vi "q2 binary to decimal.vi"() -> ()   [LabVIEW 2025]
panel:
  out "decimal":dbl
  in  "position 1":dbl
  in  "position 3":dbl
  in  "position 2":dbl
  in  "position 0":dbl
  in  "b0":bool
  in  "b1":bool
  in  "b2":bool
  in  "b3":bool
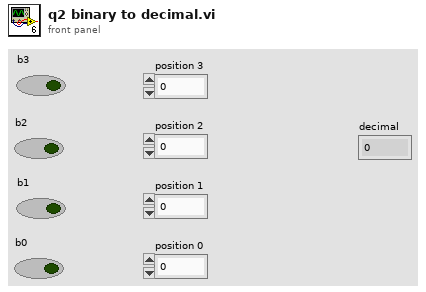
[diagram p1: front panel]
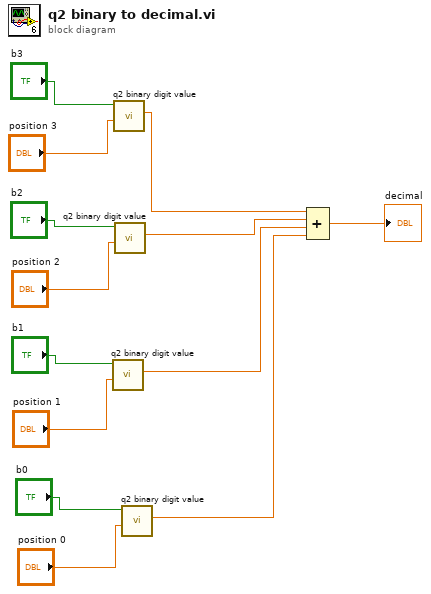
[diagram p0: block diagram]
diagram:
  n1 = call "q2 binary digit value.vi"("position"="position 1", "b"="b1") -> ("value"=w3:dbl)  [unwired: 9 in]
  n2 = call "q2 binary digit value.vi"("position"="position 3", "b"="b3") -> ("value"=w5:dbl)  [unwired: 9 in]
  n3 = call "q2 binary digit value.vi"("position"="position 2", "b"="b2") -> ("value"=w4:dbl)  [unwired: 9 in]
  n4 = call "q2 binary digit value.vi"("position"="position 0", "b"="b0") -> ("value"=w2:dbl)  [unwired: 9 in]
  n5 = Compound Arithmetic op=ADD(w5, w4, w3, w2) -> (→"decimal":dbl)
